vi "PTSequencer.await delay.vi"(0 "i ref in":refnum<vi>, 5 "error in (no error)":errorcluster) -> (14 "i ref out":refnum<vi>, 16 "next step":string, 19 "error out":errorcluster)   [LabVIEW 2014, in "PTSequencer.lvlib"]
uses:
  PTSequencer.lvlib
  CSCore/BaseSM/BaseSM.lvlib
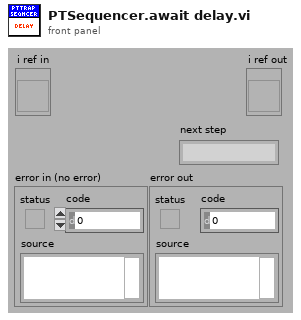
[diagram p1: front panel]
types:
  T1 = typedef "PTSequencer.lvlib/PTSequencer.i attribute.ctl" = cluster{"subsequence":bool, "mode":T2, "i step":i32, "nofLoops":i32, "i loop":i32, "Running":bool, "Paused":bool, "step done":bool, "loop done":bool, "seq done":bool, "DIM IDs":cluster{"step done":i32, "loop done":i32, "seq done":i32, "i step":i32, "i loop":i32}, "use stop conditions":bool, "stop conditions":T3[], "Step List":T5[], "DIM subsriptions":string[], "stop cond indexes":i32[], "step cond indexes":cluster{"step condition IDs":cluster{"step ID":i32, "condition ID":i32}[]}[], "Delay Start Time":timestamp, "status":string, "stopping":bool}
  T2 = typedef "PTSequencer.lvlib/PTSequencer.mode.ctl" = enum16{"single", "loop", "for loop"}
  T3 = typedef "PTSequencer.lvlib/PTSequencer.DIM service condition.ctl" = cluster{"DIM service":string, "descr":string, "nomValue":T4, "actValue":T4, "matched":bool, "DIM Status":cluster{"no link":bool, "quality":i32, "Time Stamp":timestamp}}
  T4 = typedef "CoreDefs.rawDataType.ctl" = i8[]
  T5 = typedef "PTSequencer.lvlib/PTSequencer.step.ctl" = cluster{"description":string, "object parameters":cluster{"object":string, "selector":string, "descriptor":string, "data":T4, "subsequence":bool, "call mode":enum16{"Simple DIM", "Synchronous"}, "data in":T4}, "result action":cluster{"check":bool, "passed":enum16{"Next", "Previous", "Repeat", "Jump"}, "failed":enum16{"Next", "Previous", "Repeat", "Jump"}, "jumpID_passed":i32, "jumpID_failed":i32}, "conditions":T3[], "fulfilled ":bool, "use delay":bool, "delay time (s)":dbl, "ID":i32}
  T6 = typedef "BaseSM.lvlib/BaseSM.i attribute.ctl" = cluster{"stateError":i32, "stateStatus":string, "stateQuality":T7, "ProcStateRef":refnum<vi>, "thread ref":refnum<vi>, "actState":string, "reqState":string, "SMQueue":refnum<queue>, "stateErrorID":i32, "stateStatusID":i32}
  T7 = typedef "BaseSM.lvlib/BaseSM.stateQuality.ctl" = i16
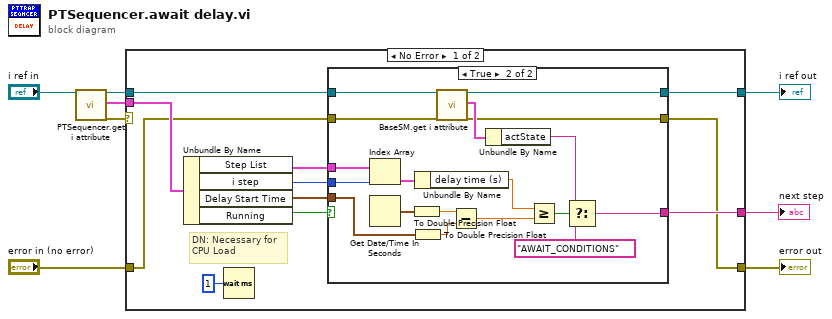
[diagram p0: block diagram]
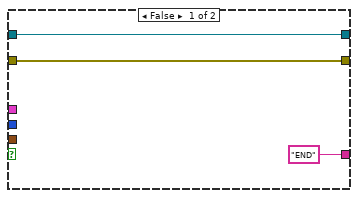
[diagram p2: hidden frame]
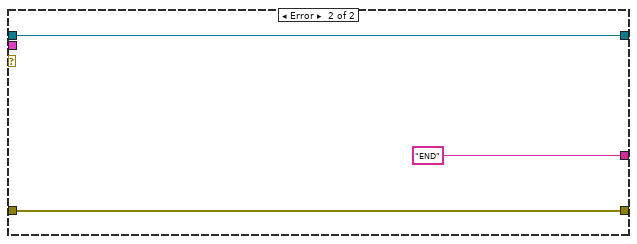
[diagram p3: hidden frame]
diagram:
  n1 = call "PTSequencer.get i attribute.vi"("i ref in"="i ref in") -> ("i ref out"=w4:refnum<vi>, "i attribute"=w5:T1, "error out"=w6:errorcluster)  [unwired: 16 in]
  n2 = case shown="No Error" w6 {
    tunnel: [w16 "END" ("actState")] -> w8
    tunnel: w5 -> [w15 _]
    tunnel: w4 -> [w14 w42]
    tunnel: [w13 w42] -> w3
    tunnel: "error in (no error)" -> [w12 w41]
    tunnel: [w11 w41] -> w1
    frame No Error {
      # "DN: Necessary for\nCPU Load"
      n3 = Unbundle By Name(w15) -> ("Step List"=w19:T5[], "i step"=w18:i32, "Delay Start Time"=w17:timestamp, "Running"=w10:bool)
      n4 = Wait (ms)(milliseconds to wait=u32 1) -> ()  [unwired: 1 out]
      n5 = case shown="True" w10 {
        tunnel: w19 -> [_ w40]
        tunnel: w18 -> [_ w39]
        tunnel: w17 -> [_ w27]
        tunnel: ["END" ("actState") w33] -> w16
        tunnel: w14 -> [w22 w32]
        tunnel: [w22 w31] -> w13
        tunnel: w12 -> [w21 w30]
        tunnel: [w21 w29] -> w11
        frame False {
        }
        frame True {
          n6 = Index Array(array=w40, index=w39) -> (element=w38:T5)
          n7 = Get Date/Time In Seconds() -> (seconds since 1Jan1904=w28:timestamp)
          n8 = To Double Precision Float(number=w28) -> (double precision float=w26:dbl)
          n9 = To Double Precision Float(number=w27) -> (double precision float=w25:dbl)
          n10 = Unbundle By Name(w38) -> ("delay time (s)"=w24:dbl)
          n11 = call "BaseSM.get i attribute.vi"("i ref in"=w32, "error in (no error)"=w30) -> ("i ref out"=w31:refnum<vi>, "i attribute"=w36:T6, "error out"=w29:errorcluster)  [unwired: 15 in]
          n12 = Subtract(x=w26, y=w25) -> (x-y=w23:dbl)
          n13 = Unbundle By Name(w36) -> ("actState"=w35:string)
          n14 = Greater Or Equal?(x=w24, y=w23) -> (x >= y?=w37:bool)
          n15 = Select(t=w35, s=w37, f="AWAIT_CONDITIONS") -> (s? t:f=w33:string)
        }
      }
    }
    frame Error {
    }
  }
  "error out" <- w1
  "i ref out" <- w3
  "next step" <- w8
